vi "LCAIO Read Status.vi"(8 "error in (no error)":errorcluster caption="Fehler (Eingang, kein Fehler)", 11 "Channel Handle":i64) -> (0 "error out":errorcluster caption="Fehler (Ausgang)", 3 "Statusword":u32)   [LabVIEW 2021, in "labbCAN_AnalogIO_API.lvlib"]
doc: "LCAIO_Func long LCAIO_CALL LCAIO_ReadStatus(dev_hdl InChanHdl, unsigned long *pdwStatus);"
uses:
  labbCAN_AnalogIO_API.lvlib
  labbCAN_AnalogIO_API.dll
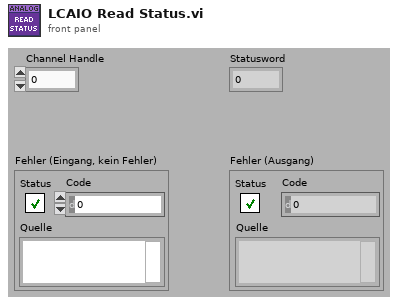
[diagram p1: front panel]
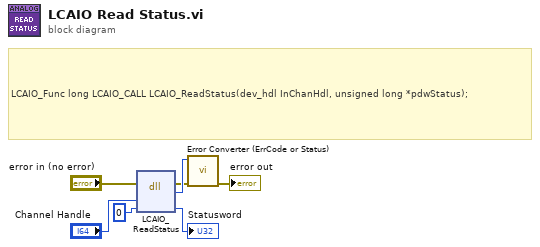
[diagram p0: block diagram]
diagram:
  # "LCAIO_Func long LCAIO_CALL LCAIO_ReadStatus(dev_hdl InChanHdl, unsigned long *pdwStatus);"
  n1 = dll-call lib="C:/Users/olaja/AppData/Local/CETONI_SDK/labbCAN_AnalogIO_API.*" fn="LCAIO_ReadStatus"(error in="error in (no error)", "Channel Handle"="Channel Handle", "Statusword"=u32 0) -> (error out=w2:errorcluster, "Rückgabetyp"=w3:i32, "Statusword"=→"Statusword":u32)  [unwired: 3 in, 1 out]
  n2 = call "Error Converter (ErrCode or Status).vi"("error in (no error)"=w2, "error code"=w3) -> ("error out"=→"error out":errorcluster)  [unwired: 9 in]
